vi "GLdrv_Close.vi"(0 "Connection ID Out":T1, 11 "error in (no error)":errorcluster) -> (15 "error out":errorcluster)   [LabVIEW 2017, in "GL860_Driver.lvlib"]
uses:
  GL860_Driver.lvlib
  ConnectionID.ctl
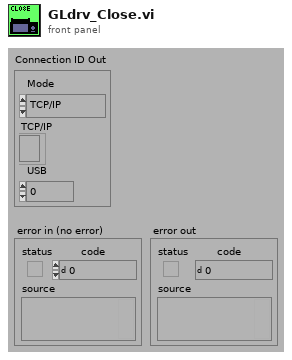
[diagram p1: front panel]
types:
  T1 = typedef "ConnectionID.ctl" = cluster{"Mode":enum16{"TCP/IP", "USB"}, "TCP/IP":refnum<k5>, "USB":i32}
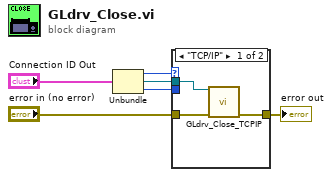
[diagram p0: block diagram]
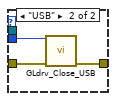
[diagram p2: hidden frame]
diagram:
  n1 = Unbundle("Connection ID Out") -> ("Mode"=w2:enum16{"TCP/IP", "USB"}, "TCP/IP"=w5:refnum<k5>, "USB"=w1:i32)
  n2 = case shown="\"TCP/IP\"" w2 {
    tunnel: w5 -> [w9 _]
    tunnel: "error in (no error)" -> [w8 w11]
    tunnel: [w7 w10] -> w3
    tunnel: w1 -> [_ w12]
    frame "TCP/IP" {
      n3 = call "GLdrv_Close_TCPIP.vi"("connection ID"=w9, "error in (no error)"=w8) -> ("error out"=w7:errorcluster)  [unwired: 13 out]
    }
    frame "USB" {
      n4 = call "GLdrv_Close_USB.vi"("hDevice"=w12, "error in (no error)"=w11) -> ("error out"=w10:errorcluster)  [unwired: 13 out]
    }
  }
  "error out" <- w3
